vi "Actor Core.vi"(8 "error in":errorcluster, 11 "New Session in":refnum<class "New Session.lvclass">) -> (0 "error out":errorcluster, 3 "Actor out":refnum<class "Actor.lvclass">)   [LabVIEW 2014, in "New Session Class.lvlib" / "New Session.lvclass"]
doc: "(<B>Filename</B>: Actor Framework.lvlib:Actor.lvclass:Actor Core.vi)\n\nReceives messages to the actor, reacts to them, and initiates any error handling that may shut the actor down.\n\nDescendant classes may override this VI to append parallel tasks for the actor to complete while it handles messages. Overrides use the Call Parent Method node."
uses:
  New Session.lvclass
  <vilib>/ActorFramework/Actor/Actor.lvclass
  Subpanel Insertion/Subpanel Inserter.lvclass
panel:
  out "i":i32
  out "stop value":bool
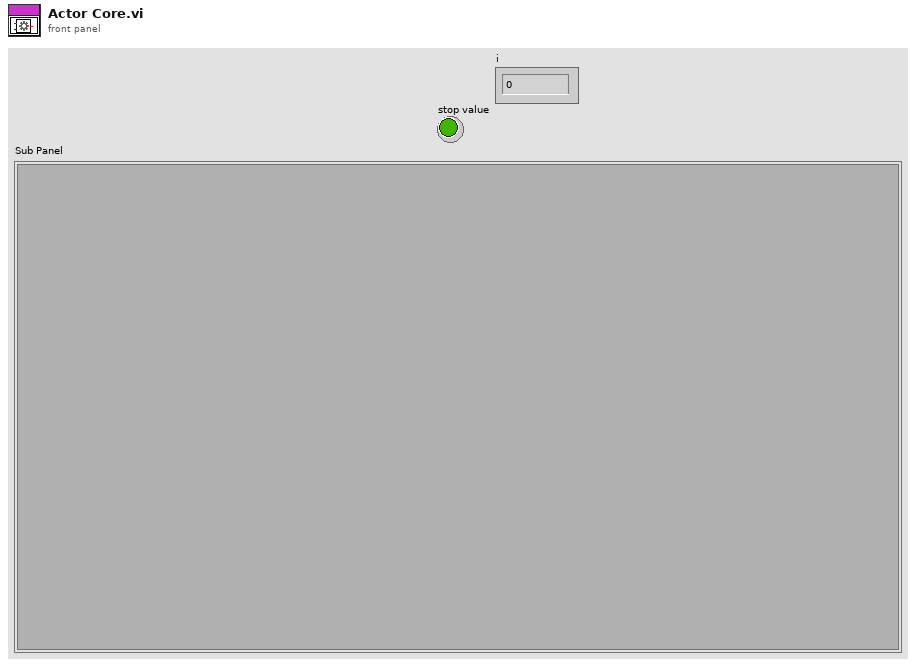
[diagram p1: front panel]
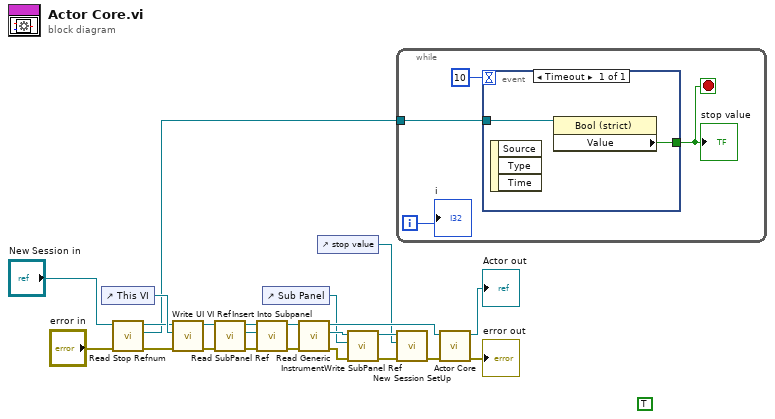
[diagram p0: block diagram]
diagram:
  (unwired) TRUE ("Value (Signaling)")
  n1 = control-ref of="This VI"() -> (w14:refnum<vi>)
  n2 = call-dynamic "Read Stop Refnum.vi"("error in (no error)"="error in", "New Session in"="New Session in") -> ("error out"=w2:errorcluster, "Stop Refnum"=w1:refnum<vi>, "New Session out"=w3:refnum<class "New Session.lvclass">)  [unwired: 7 in]
  n3 = call-dynamic "Write UI VI Ref.vi"("error in (no error)"=w2, "UI VI Ref"=w14, "Subpanel Inserter in"=w3) -> ("error out"=w7:errorcluster, "Subpanel Inserter out"=w8:refnum<class "New Session.lvclass">)  [unwired: 7 in]
  n4 = call-dynamic "Read SubPanel Ref.vi"("error in (no error)"=w7, "Subpanel Inserter in"=w8) -> ("error out"=w12:errorcluster, "SubPanel Ref"=w11:refnum<vi>, "Subpanel Inserter out"=w13:refnum<class "New Session.lvclass">)  [unwired: 7 in]
  n5 = call "Insert Into Subpanel.vi"("Error In"=w12, "SubPanel Ref"=w11, "Subpanel Inserter"=w13) -> ("error out"=w9:errorcluster, "Subpanel Inserter"=w10:refnum<class "New Session.lvclass">)  [unwired: 7 in]
  n6 = control-ref of="Sub Panel"() -> (w18:refnum<vi>)
  n7 = call-dynamic "Read Generic Instrument.vi"("error in (no error)"=w9, "New Session in"=w10) -> ("error out"=w16:errorcluster, "Subpanel Insertion.lvlib:Subpanel Inserter.lvclass"=w19:refnum<class "Subpanel Inserter.lvclass">, "New Session out"=w20:refnum<class "New Session.lvclass">)  [unwired: 7 in]
  n8 = control-ref of="stop value"() -> (w6:refnum<vi>)
  n9 = call-dynamic "Write SubPanel Ref.vi"("error in (no error)"=w16, "SubPanel Ref"=w18, "Subpanel Inserter in"=w19) -> ("error out"=w15:errorcluster, "Subpanel Inserter out"=w17:refnum<class "Subpanel Inserter.lvclass">)  [unwired: 7 in]
  n10 = while {
    tunnel: w1 -> [w25]
    i -> [w24]
    stop <- w26 stop-if-true
    n11 = event shown="[0] Timeout" {
      selector: _ -> [_]
      dyn-events: _ -> [_]
      timeout: 10 -> [_]
      tunnel: [w28] -> w26
      tunnel: w25 -> [w29]
      event Timeout {
        n12 = event-data() -> ()  [unwired: 1 in, 3 out]
        n13 = property class="Bool (strict)"(reference=w29) -> ("Value"=w28:bool)  [unwired: 1 in, 2 out]
      }
    }
    "stop value" <- w26
    "i" <- w24
  }
  n14 = call-dynamic "New Session SetUp.vi"("error in (no error)"=w15, "Stop Refnum"=w6, "Subpanel Inserter in"=w17) -> ("error out"=w21:errorcluster)  [unwired: 7 in, 1 out]
  n15 = call-parent "Actor Core.vi"("error in"=w21, "Actor in"=w20) -> ("error out"=→"error out":errorcluster, "Actor out"=→"Actor out":refnum<class "Actor.lvclass">)  [unwired: 8 in]
